vi "EF_EnQError.vi"(8 "error in (no error)":errorcluster, 11 "Queue in":T1) -> ()   [LabVIEW 2017]
uses:
  Types/EF_DAQThread_QRef.ctl
  Types/EF_DAQThread_QData.ctl
  Types/EF_DAQThread_QCmds.ctl
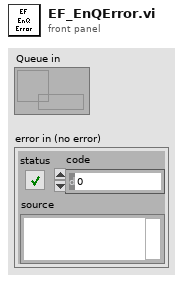
[diagram p1: front panel]
types:
  T1 = typedef "EF_DAQThread_QRef.ctl" = refnum<queue>
  T2 = typedef "EF_DAQThread_QCmds.ctl" = enum16{"Idle", "Init", "InitHW", "SetCFD0", "SetCFD1", "SetCh0Divider", "SetCh0Offset", "SetOffset", "SetBinning", "GetResolution", "GetRates", "StartMeas", "ReadFiFo", "StopMeas", "WriteStatus", "_Error_", "Exit"}
  T3 = typedef "EF_DAQThread_QData.ctl" = cluster{"EF_DAQThread_Cmds":T2, "Parameter":i32[], "error in (no error)":errorcluster}
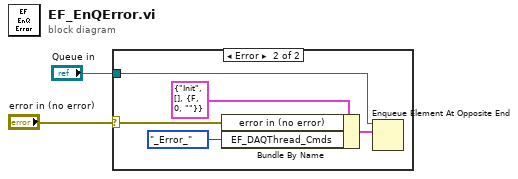
[diagram p0: block diagram]
diagram:
  n1 = case shown="Error" "error in (no error)" {
    selector: "error in (no error)" -> [_ w5]
    tunnel: "Queue in" -> [_ w7]
    frame No Error {
    }
    frame Error {
      n2 = Bundle By Name(cluster=T3 {"EF_DAQThread_Cmds"=enum."Init", "Parameter"=[], "error in (no error)"={"status"=FALSE, "code"=0, "source"=""}} ("element"), "error in (no error)"=w5, "EF_DAQThread_Cmds"=EF_DAQThread_QCmds."_Error_") -> (w3:T3)
      n3 = Enqueue Element At Opposite End(queue=w7, element=w3) -> ()  [unwired: 2 in, 3 out]
    }
  }
